vi "TDMS Write Events Data_Kafka.vi"() -> ()   [LabVIEW 2019]
doc: "This example demonstrates how to write measured data along with text and timestamp values to a .tdms file using the TDMS API. TDMS files written by this example can be read by the example TDMS Read Events Data.vi."
panel:
  in  "Stop":bool
  out "Measured Data":waveform(dbl)[](graph)
  # "Overview: Demonstrates the use of the TDMS Write function to write measured data along with text and timestamp values to a .tdms file.\nInstructions:\n1. Run the VI.\n2. Click Stop to stop the VI.\n3. Open the TDMS Read Events Data.vi example to view the data generated by this VI."
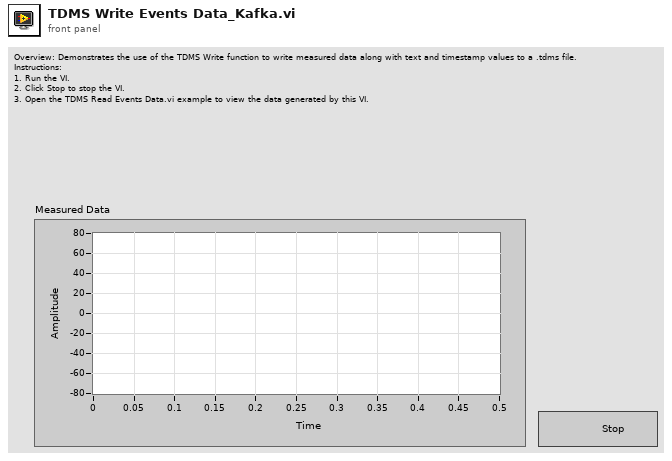
[diagram p1: front panel]
types:
  T1 = enum16{"open", "open or create", "create or replace", "create", "open (read-only)"}
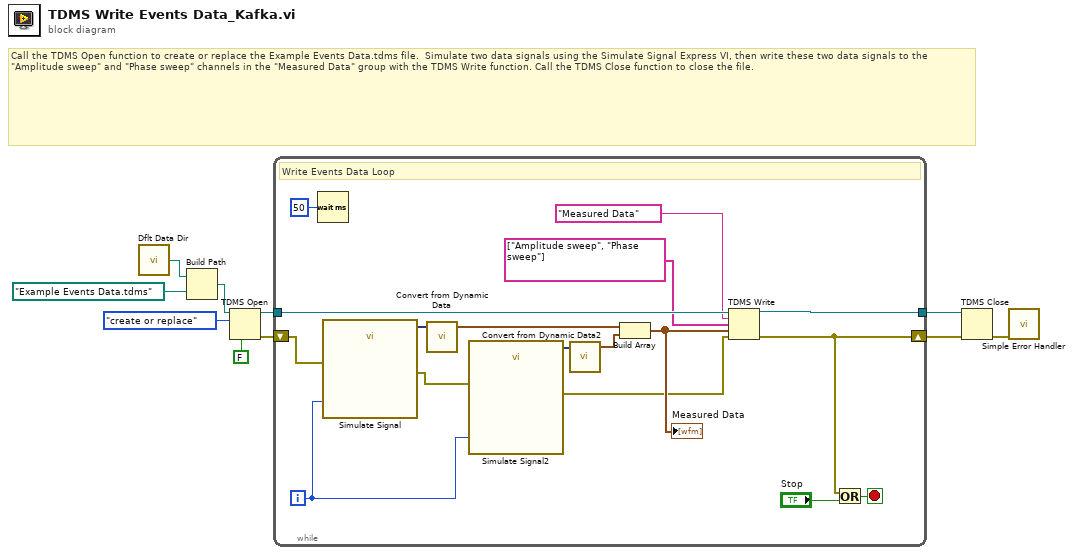
[diagram p0: block diagram]
diagram:
  # "Call the TDMS Open function to create or replace the Example Events Data.tdms file.  Simulate two data signals using the Simulate Signal Express VI, then write these two data signals to the \"Amplitude sweep\" and \"Phase sweep\" channels in the \"Measured Data\" group with the TDMS Write function. Call the TDMS Close function to close the file."
  n1 = call <vilib>:"Dflt Data Dir.vi"() -> ("App:Default Data Directory"=w10:path)
  n2 = Build Path(base path=w10, name or relative path=path "Example Events Data.tdms" ("file path")) -> (appended path=w3:path)
  n3 = TDMS Open(6:FALSE ("disable buffering (T)"), 10:T1."create or replace" ("operation"), 11:w3) -> (0:w6:errorcluster, 3:w7:refnum<k34>)  [unwired: 4 in]
  n4 = while {
    shift-right: [w11] -> w4
    shift-left: w6 -> [w24]
    tunnel: w7 -> [w17]
    tunnel: [w12] -> w5
    i -> [w21]
    stop <- w25 stop-if-true
    # "Write Events Data Loop"
    n5 = Wait (ms)(milliseconds to wait=u32 50) -> ()  [unwired: 1 out]
    n6 = call "Simulate Signal"("Amplitude"=w21, "error in (no error)"=w24) -> ("Sine"=w23:dynamicdata, "error out"=w22:errorcluster)  [unwired: 12 in]
    n7 = call "Convert from Dynamic Data"("Dynamic Data Type"=w23) -> ("Waveform"=w18:waveform(dbl))  [unwired: 3 in]
    n8 = call "Simulate Signal2"("Phase"=w21, "error in (no error)"=w22) -> ("Sine"=w20:dynamicdata, "error out"=w13:errorcluster)  [unwired: 12 in]
    n9 = call "Convert from Dynamic Data2"("Dynamic Data Type"=w20) -> ("Waveform"=w19:waveform(dbl))  [unwired: 3 in]
    n10 = Build Array(w18, w19) -> (w14:waveform(dbl)[])
    "Measured Data" <- w14
    n11 = TDMS Write(0:w17, 5:"Measured Data" ("group name"), 7:string[] ["Amplitude sweep", "Phase sweep"] ("channel names"), 9:w14, 11:w13) -> (4:w12:refnum<k34>, 15:w11:errorcluster)  [unwired: 1 in, 2 out]
    n12 = Or(x=w11, y="Stop") -> (x .or. y?=w25:bool)
  }
  n13 = TDMS Close(8:w4, 11:w5) -> (0:w1:errorcluster)  [unwired: 1 out]
  n14 = call <vilib>:"Simple Error Handler.vi"("error in (no error)"=w1) -> ()  [unwired: 2 in, 7 out]
